vi "instantiate_webpage_datasource.vi"(0 "webpages":string[](array[string]), 11 "error in (no error)":errorcluster) -> (4 "datasource_webpage out":refnum<class "datasource_webpage.lvclass">, 15 "error out":errorcluster)   [LabVIEW 2020, in "datasource_webpage.lvclass"]
uses:
  datasource_webpage.lvclass
  datasource_webpage.lvclass/datasource_webpage.ctl
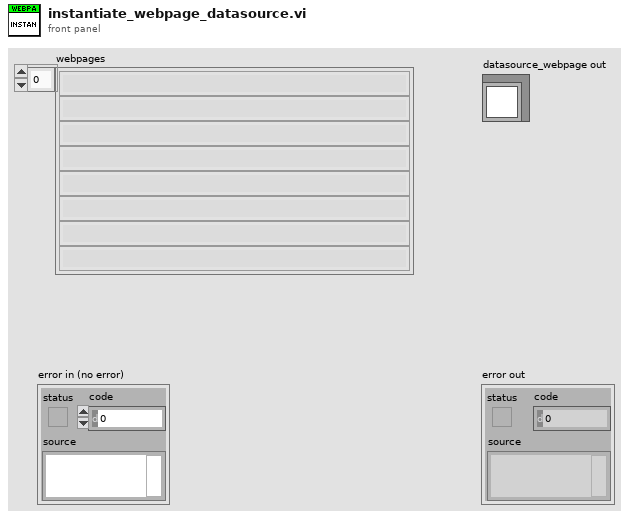
[diagram p1: front panel]
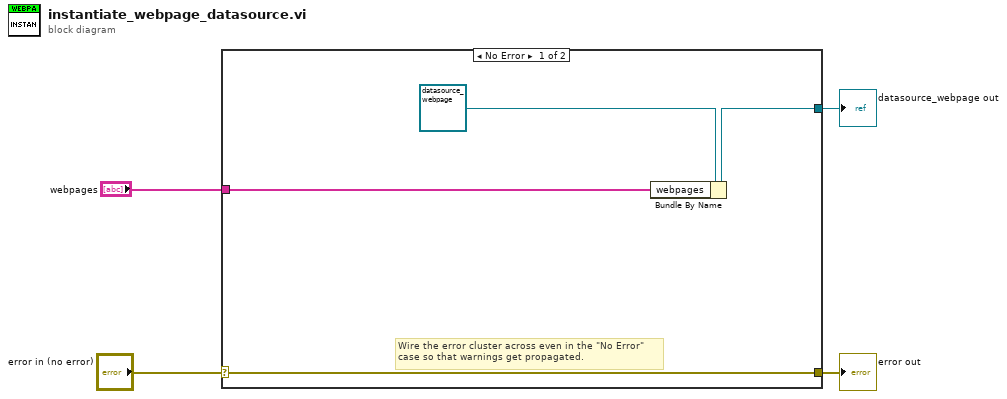
[diagram p0: block diagram]
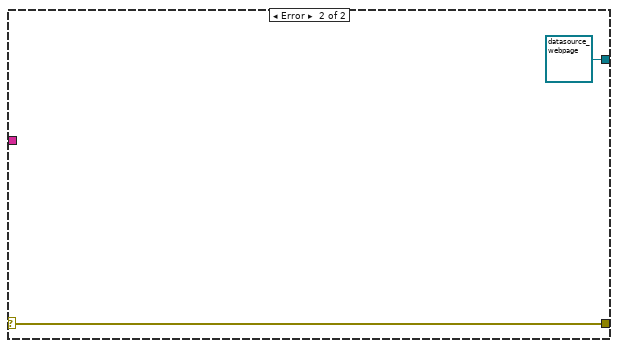
[diagram p2: hidden frame]
diagram:
  n1 = case shown="No Error" "error in (no error)" {
    selector: "error in (no error)" -> [w8 w10]
    tunnel: [w8 w10] -> w3
    tunnel: [w6 refnum<class "datasource_webpage.lvclass"> refnum ("datasource_webpage out")] -> w2
    tunnel: "webpages" -> [w5 _]
    frame No Error {
      # "Wire the error cluster across even in the \"No Error\"\ncase so that warnings get propagated."
      n2 = Bundle By Name(cluster=refnum<class "datasource_webpage.lvclass"> refnum ("datasource_webpage out"), "webpages"=w5) -> (w6:refnum<class "datasource_webpage.lvclass">)
    }
    frame Error {
    }
  }
  "error out" <- w3
  "datasource_webpage out" <- w2
